vi "Pack Step Value.vi"(8 "error in":errorcluster, 10 "Value":string, 11 "Switch DBL in":refnum<class "Switch DBL.lvclass">) -> (0 "error out":errorcluster, 3 "Switch DBL out":refnum<class "Switch DBL.lvclass">)   [LabVIEW 2016, in "Sequence Composition.lvlib" / "Switch DBL.lvclass"]
uses:
  Switch DBL.lvclass
  Switch DBL.lvclass/Switch DBL.ctl
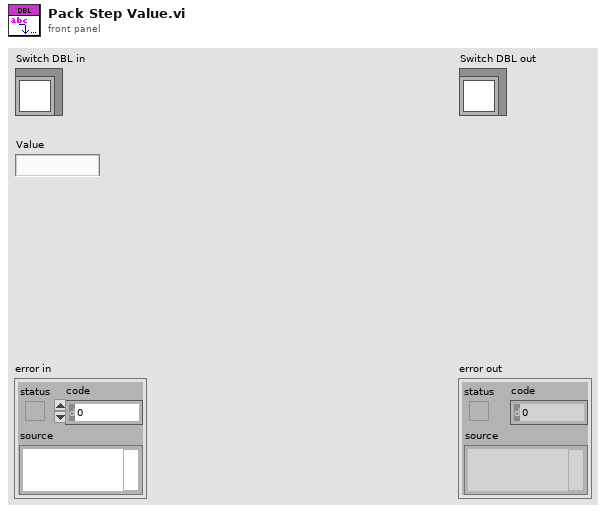
[diagram p1: front panel]
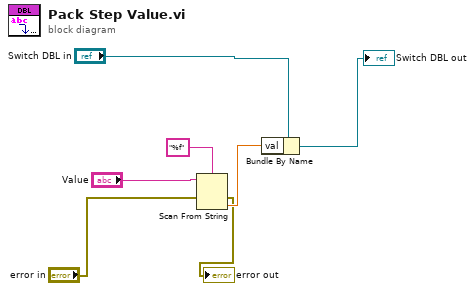
[diagram p0: block diagram]
diagram:
  n1 = Scan From String(format string="%f", input string="Value", error in="error in") -> (error out=→"error out":errorcluster, output 1=w3:dbl)  [unwired: 2 in, 2 out]
  n2 = Bundle By Name(cluster="Switch DBL in", "val"=w3) -> (→"Switch DBL out":refnum<class "Switch DBL.lvclass">)
